vi "SetBaseClasses.vi"(0 "ClassReader in":refnum<class "ClassReader.lvclass">, 1 "Inheritance":path[](array[path]), 5 "error in (no error)":errorcluster) -> (14 "ClassReader out":refnum<class "ClassReader.lvclass">, 19 "error out":errorcluster)   [LabVIEW 2016, in "ClassReader.lvclass"]
uses:
  <resource>/Framework/Providers/Open_GDS/ClassProviders/Provider_BaseClassInterface/ClassReader_class/ClassReader.lvclass
  <resource>/Framework/Providers/Open_GDS/ClassProviders/Provider_BaseClassInterface/ClassReader_class/ClassReader.lvclass/ClassReader.ctl
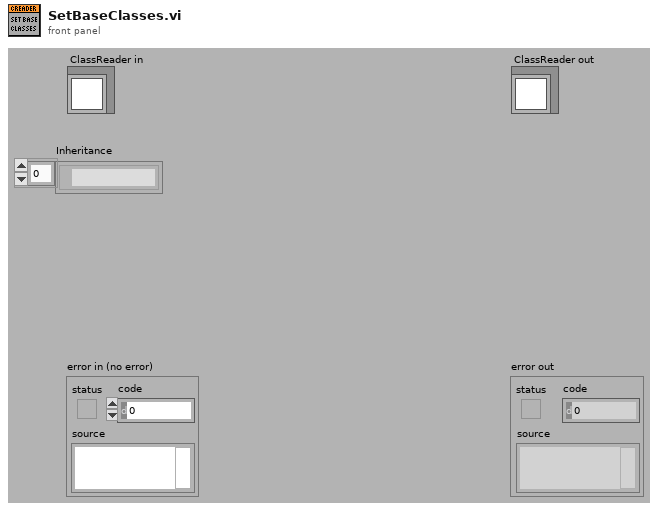
[diagram p1: front panel]
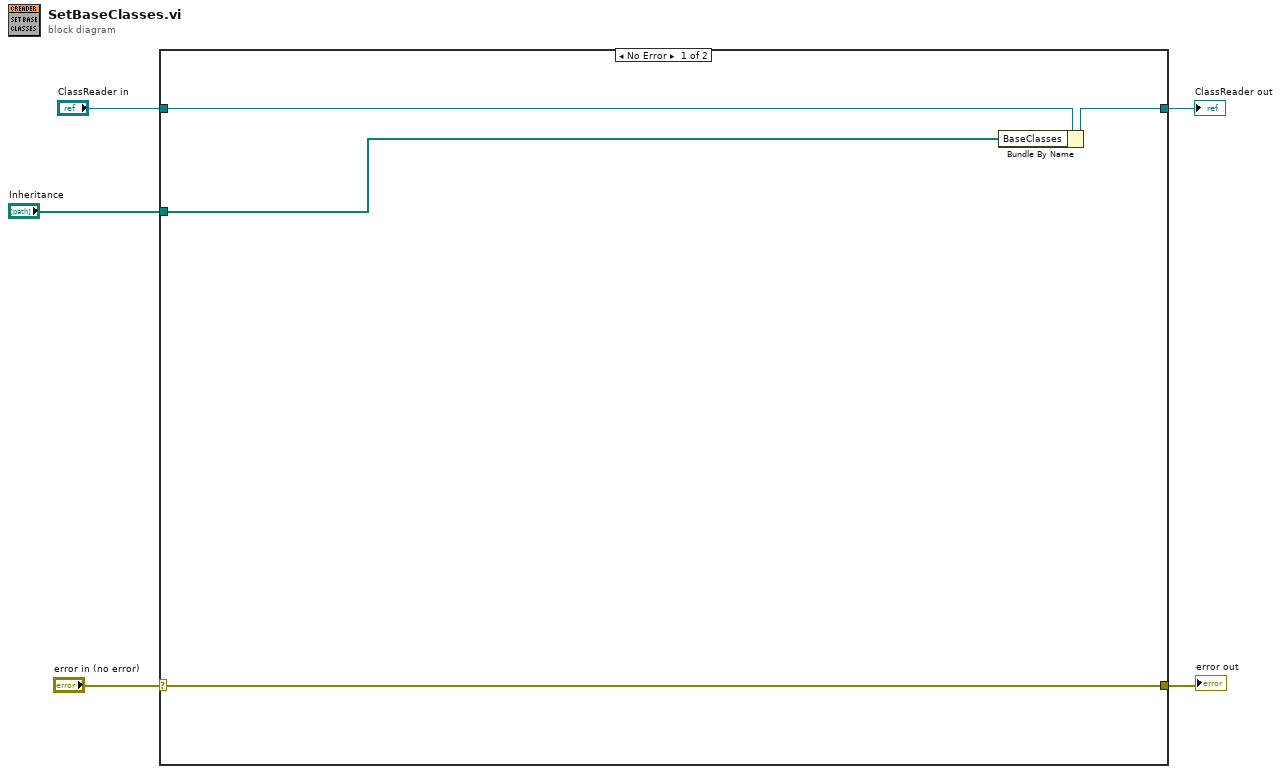
[diagram p0: block diagram]
diagram:
  n1 = case shown="No Error" "error in (no error)" {
    selector: "error in (no error)" -> [w6 w11]
    tunnel: [w6 w11] -> w4
    tunnel: [w8 w10] -> w2
    tunnel: "ClassReader in" -> [w9 w10]
    tunnel: "Inheritance" -> [w7 _]
    frame No Error {
      n2 = Bundle By Name(cluster=w9, "BaseClasses"=w7) -> (w8:refnum<class "ClassReader.lvclass">)
    }
    frame Error {
    }
  }
  "error out" <- w4
  "ClassReader out" <- w2
